vi "IV programa 1_1.vi"() -> ()   [LabVIEW 2020]
panel:
  in  "stop":bool
  out "btn 6":bool
  out "btn 5":bool
  out "btn 4":bool
  out "btn 3":bool
  out "btn 2":bool
  out "btn 1":bool
  in  "boton 6":bool
  in  "boton 5":bool
  in  "boton 4":bool
  in  "boton 3":bool
  in  "boton 2":bool
  in  "boton 1":bool
  # "1.1: Elabore un programa donde muestre un ejemplo de cada uno de los modos de acción mecánica de\nlos botones (6 modos). considere que deberá ser claro de comprender para el usuario."
  # "swith when pressed ==>"
  # "swith when relased  ==>"
  # "swith until relased  ==>"
  # "latch when pressed  ==>"
  # "latch when relaced  ==>"
  # "latch until relaced  ==>"
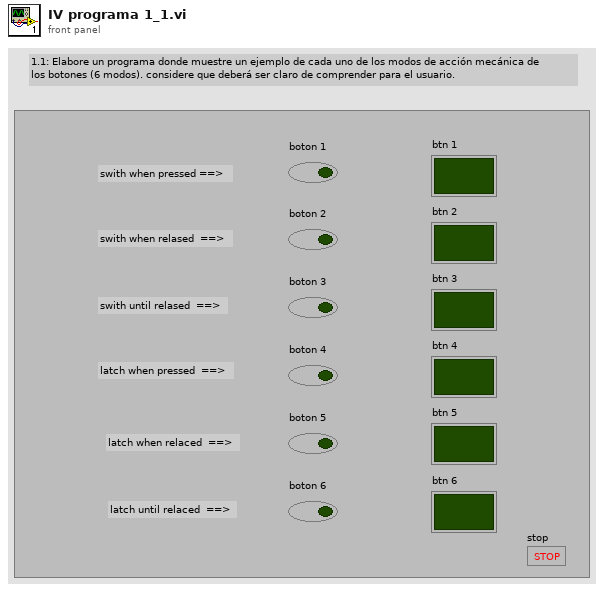
[diagram p1: front panel]
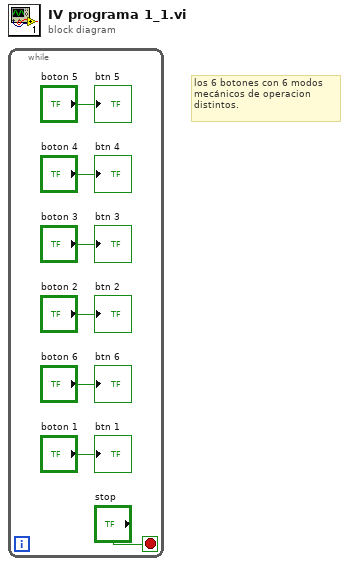
[diagram p0: block diagram]
diagram:
  # "los 6 botones con 6 modos \nmecánicos de operacion \ndistintos."
  n1 = while {
    stop <- "stop" stop-if-true
    "btn 1" <- "boton 1"
    "btn 2" <- "boton 2"
    "btn 3" <- "boton 3"
    "btn 4" <- "boton 4"
    "btn 5" <- "boton 5"
    "btn 6" <- "boton 6"
  }
